vi "SMU_development_test.vi"() -> ()   [LabVIEW 2018]
uses:
  InstrControl/SupplyControl/SupplyControl.lvclass
  InstrControl/InstrControl.lvclass
  <instrlib>/Keithley 2600 Series/Keithley 2600 Series.lvlib
  InstrControl/InstrumentSetup.vi
panel:
  in  "Instrument name IN":string(combo)="Keithley 2657"
  in  "No. of measurements":i32=10
  out "Waveform Chart":dbl(graph)=7.46136e-05
  out "Current Voltage 2":dbl format="%.2f"
  out "Compliance exceeded":bool
  out "Current Voltage":dbl=5.0 format="%.2f"
  out "Instrument name OUT":string="Keithley 2657A"
  out "Current in nA":dbl=7.46136e-05 format="%#.6g"
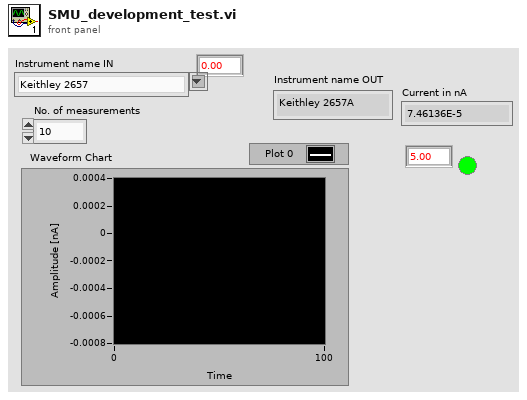
[diagram p1: front panel]
types:
  T1 = enum16{"Supply", "LCR", "Multimeter", "Switching"}
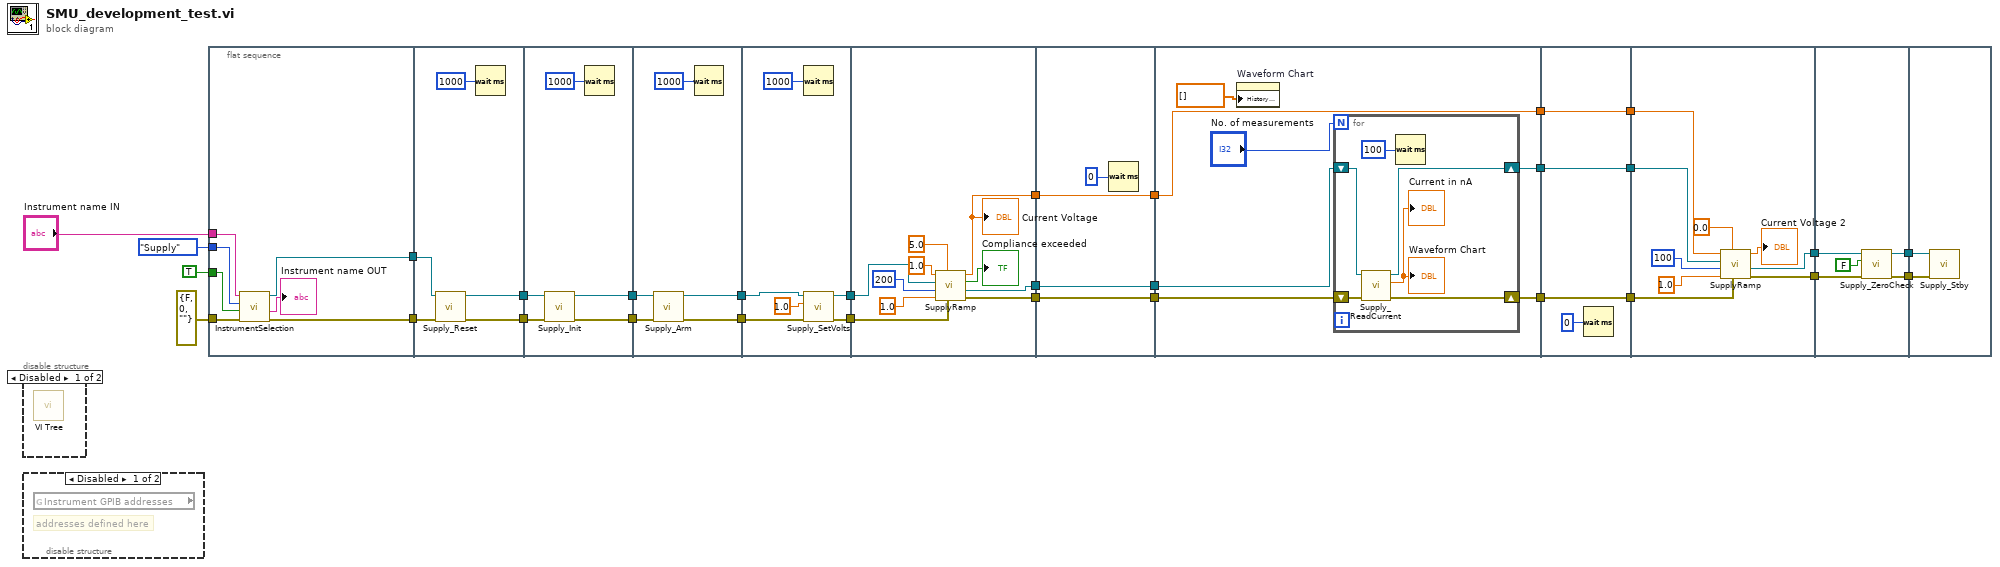
[diagram p0: block diagram]
diagram:
  n1 = disable-structure shown="Disabled" {
    frame Disabled {
      n2 = call <instrlib>:"VI Tree.vi"() -> ()  [unwired: 12 in]
    }
    frame Enabled {
    }
  }
  n3 = disable-structure shown="Disabled" {
    frame Disabled {
      # "addresses defined here"
      n4 = global read "InstrumentSetup.vi" "Instrument GPIB addresses"() -> ()  [unwired: 1 out]
    }
    frame Enabled {
    }
  }
  n5 = flat-sequence {
    tunnel: errorcluster {"status"=FALSE, "code"=0, "source"=""} ("error in (no error)") -> [w36]
    tunnel: TRUE ("Verify GPIB address") -> [w35]
    tunnel: T1."Supply" ("Instrument type") -> [w34]
    tunnel: [w33] -> w25
    tunnel: [w32] -> w24
    tunnel: "Instrument name IN" -> [w31]
    tunnel: [w40] -> w27
    tunnel: [w39] -> w26
    tunnel: w25 -> [w42]
    tunnel: w24 -> [w41]
    tunnel: w27 -> [w47]
    tunnel: w26 -> [w46]
    tunnel: [w45] -> w23
    tunnel: [w44] -> w22
    tunnel: w23 -> [w51]
    tunnel: [w49] -> w21
    tunnel: w22 -> [w52]
    tunnel: [w50] -> w20
    tunnel: w21 -> [w56]
    tunnel: [w54] -> w19
    tunnel: w20 -> [w57]
    tunnel: [w55] -> w18
    tunnel: w19 -> [w67]
    tunnel: w18 -> [w68]
    tunnel: [w61] -> w6
    tunnel: [w60] -> w4
    tunnel: [w59] -> w2
    tunnel: w6 -> [w72]
    tunnel: [w72] -> w5
    tunnel: w4 -> [w71]
    tunnel: [w71] -> w3
    tunnel: w2 -> [w70]
    tunnel: [w70] -> w1
    tunnel: w5 -> [w78]
    tunnel: w3 -> [w79]
    tunnel: [w76] -> w12
    tunnel: [w75] -> w10
    tunnel: w1 -> [w74]
    tunnel: [w74] -> w8
    tunnel: w12 -> [w89]
    tunnel: [w89] -> w11
    tunnel: w10 -> [w88]
    tunnel: [w88] -> w9
    tunnel: w8 -> [w87]
    tunnel: [w87] -> w7
    tunnel: w11 -> [w98]
    tunnel: w9 -> [w97]
    tunnel: w7 -> [w93]
    tunnel: [w91] -> w17
    tunnel: [w90] -> w15
    tunnel: w17 -> [w101]
    tunnel: [w100] -> w16
    tunnel: w15 -> [w103]
    tunnel: [w99] -> w14
    tunnel: w16 -> [w105]
    tunnel: w14 -> [w104]
    frame #0 {
      n6 = call "InstrumentSelection.vi"("error in (no error)"=w36, "Verify GPIB address"=w35, "Instrument type"=w34, "Instrument name IN"=w31) -> ("error out"=w33:errorcluster, "Instrument name OUT"=→"Instrument name OUT":string, "Supply"=w32:refnum<class "SupplyControl.lvclass">)  [unwired: 2 in, 3 out]
    }
    frame #1 {
      n7 = call-dynamic "Supply_Reset.vi"("error in (no error)"=w42, "SupplyControl in"=w41) -> ("error out"=w40:errorcluster, "SupplyControl out"=w39:refnum<class "SupplyControl.lvclass">)  [unwired: 8 in]
      n8 = Wait (ms)(milliseconds to wait=u32 1000) -> ()  [unwired: 1 out]
    }
    frame #2 {
      n9 = call-dynamic "Supply_Init.vi"("error in (no error)"=w47, "SupplyControl in"=w46) -> ("error out"=w45:errorcluster, "SupplyControl out"=w44:refnum<class "SupplyControl.lvclass">)  [unwired: 8 in]
      n10 = Wait (ms)(milliseconds to wait=u32 1000) -> ()  [unwired: 1 out]
    }
    frame #3 {
      n11 = call-dynamic "Supply_Arm.vi"("error in (no error)"=w51, "SupplyControl in"=w52) -> ("error out"=w49:errorcluster, "SupplyControl out"=w50:refnum<class "SupplyControl.lvclass">)  [unwired: 8 in]
      n12 = Wait (ms)(milliseconds to wait=u32 1000) -> ()  [unwired: 1 out]
    }
    frame #4 {
      n13 = Wait (ms)(milliseconds to wait=u32 1000) -> ()  [unwired: 1 out]
      n14 = call-dynamic "Supply_SetVolts.vi"("error in (no error)"=w56, "Volts IN [V]"=1.0, "SupplyControl in"=w57) -> ("error out"=w54:errorcluster, "SupplyControl out"=w55:refnum<class "SupplyControl.lvclass">)  [unwired: 6 in, 1 out]
    }
    frame #5 {
      n15 = call "SupplyRamp.vi"("error in"=w67, "Requested Voltage"=5.0, "Step Size"=1.0, "Step Delay"=u32 200, "Supply IN"=w68, "Starting Voltage"=1.0) -> ("error out"=w60:errorcluster, "Supply OUT"=w61:refnum<class "SupplyControl.lvclass">, "Compliance exceeded"=→"Compliance exceeded":bool, "Current Voltage"=w59:dbl)  [unwired: 2 in]
      "Current Voltage" <- w59
    }
    frame #6 {
      n16 = Wait (ms)(milliseconds to wait=u32 0) -> ()  [unwired: 1 out]
    }
    frame #7 {
      n17 = property on="Waveform Chart" class="WFChart (strict)"("History Data"=dbl[] []) -> ()  [unwired: 2 in, 2 out]
      n18 = for {
        N: "No. of measurements" -> [_]
        shift-right: [w82] -> w76
        shift-left: w78 -> [w84]
        shift-right: [w81] -> w75
        shift-left: w79 -> [w85]
        n19 = call-dynamic "Supply_ReadCurrent.vi"("error in (no error)"=w85, "SupplyControl in"=w84) -> ("error out"=w81:errorcluster, "Current in nA"=→"Current in nA" →"Waveform Chart":dbl, "SupplyControl out"=w82:refnum<class "SupplyControl.lvclass">)  [unwired: 7 in]
        n20 = Wait (ms)(milliseconds to wait=u32 100) -> ()  [unwired: 1 out]
      }
    }
    frame #8 {
      n21 = Wait (ms)(milliseconds to wait=u32 0) -> ()  [unwired: 1 out]
    }
    frame #9 {
      n22 = call "SupplyRamp.vi"("error in"=w97, "Requested Voltage"=0.0, "Step Size"=1.0, "Step Delay"=u32 100, "Supply IN"=w98, "Starting Voltage"=w93) -> ("error out"=w90:errorcluster, "Supply OUT"=w91:refnum<class "SupplyControl.lvclass">, "Current Voltage"=→"Current Voltage 2":dbl)  [unwired: 2 in, 1 out]
    }
    frame #10 {
      n23 = call-dynamic "Supply_ZeroCheck.vi"("error in (no error)"=w103, "enable/disable"=FALSE, "SupplyControl in"=w101) -> ("error out"=w99:errorcluster, "SupplyControl out"=w100:refnum<class "SupplyControl.lvclass">)  [unwired: 7 in]
    }
    frame #11 {
      n24 = call-dynamic "Supply_Stby.vi"("error in (no error)"=w104, "SupplyControl in"=w105) -> ()  [unwired: 8 in, 2 out]
    }
  }
